vi "Keithley_6221_data.vi"() -> (0 "String":string)   [LabVIEW 2019]
uses:
  Instrument_Setup.vi
panel:
  out "String 3":string
  out "String 2":string
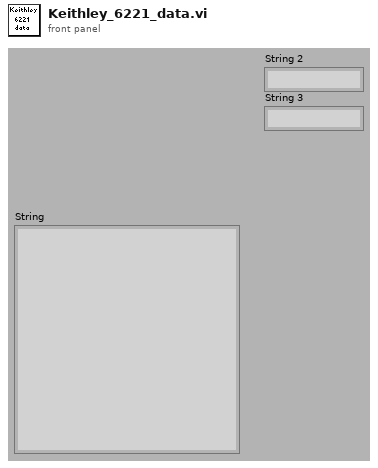
[diagram p1: front panel]
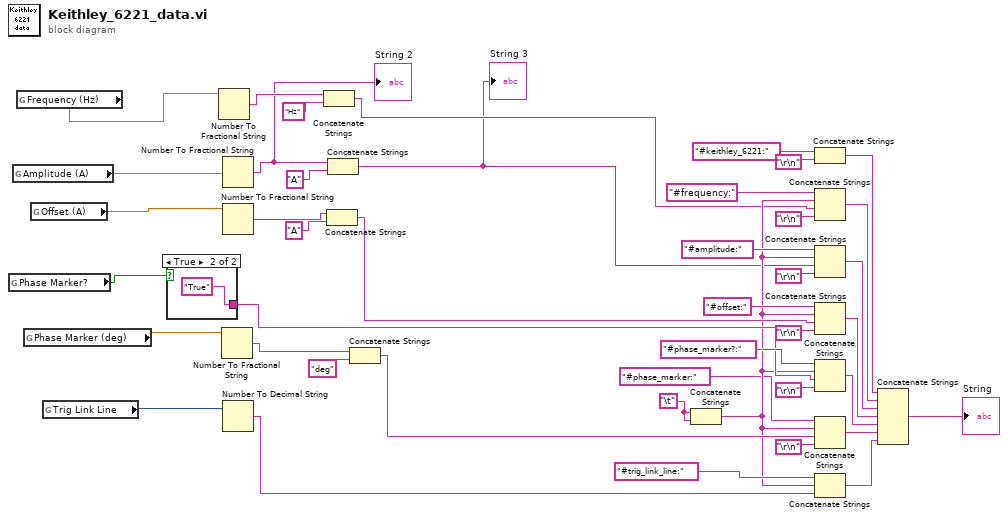
[diagram p0: block diagram]
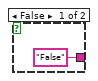
[diagram p2: hidden frame]
diagram:
  w43 = "\t"
  n1 = global read "Instrument_Setup.vi" "Phase Marker?"() -> (w20:bool)
  n2 = global read "Instrument_Setup.vi" "Amplitude (A)"() -> (w24:dbl)
  n3 = global read "Instrument_Setup.vi" "Frequency (Hz)"() -> (w1:dbl)
  n4 = global read "Instrument_Setup.vi" "Phase Marker (deg)"() -> (w22:dbl)
  n5 = global read "Instrument_Setup.vi" "Offset (A)"() -> (w23:dbl)
  n6 = global read "Instrument_Setup.vi" "Trig Link Line"() -> (w21:i32)
  n7 = case shown="True" w20 {
    tunnel: ["False" "True"] -> w19
    frame False {
    }
    frame True {
    }
  }
  n8 = Number To Fractional String(number=w1) -> (F-format string=w6:string)  [unwired: 3 in]
  n9 = Number To Fractional String(number=w22) -> (F-format string=w14:string)  [unwired: 3 in]
  n10 = Number To Fractional String(number=w24) -> (F-format string=w3:string)  [unwired: 3 in]
  "String 2" <- w3
  n11 = Number To Fractional String(number=w23) -> (F-format string=w15:string)  [unwired: 3 in]
  n12 = Number To Decimal String(number=w21) -> (decimal integer string=w10:string)  [unwired: 1 in]
  n13 = Concatenate Strings(w6, "Hz") -> (w5:string)
  n14 = Concatenate Strings(w15, "A") -> (w13:string)
  n15 = Concatenate Strings(w3, "A") -> (w2:string)
  "String 3" <- w2
  n16 = Concatenate Strings(w14, "deg") -> (w12:string)
  n17 = Concatenate Strings(w43, w43) -> (w11:string)
  n18 = Concatenate Strings("#keithley_6221:", "\r\n") -> (w28:string)
  n19 = Concatenate Strings("#frequency:", w11, w5, "\r\n") -> (w38:string)
  n20 = Concatenate Strings("#amplitude:" ("String"), w11, w2, "\r\n") -> (w39:string)
  n21 = Concatenate Strings("#offset:" ("String"), w11, w13, "\r\n") -> (w40:string)
  n22 = Concatenate Strings("#phase_marker?:" ("String"), w11, w19, "\r\n") -> (w41:string)
  n23 = Concatenate Strings("#phase_marker:" ("String"), w11, w12, "\r\n") -> (w42:string)
  n24 = Concatenate Strings("#trig_link_line:" ("String"), w11, w10) -> (w9:string)
  n25 = Concatenate Strings(w28, w38, w39, w40, w41, w42, w9) -> (→"String":string)
